vi "Disabled - Auton Script System (SubVI).vi"(8 "Alliance Color Input":string, 9 "Reload File Names":bool, 10 "Down File":bool, 11 "Up File":bool) -> (0 "error out":errorcluster, 1 "Files Reloaded":bool, 2 "Alliance Color":string, 3 "all rows":dbl[][](array[numeric]), 4 "File Name":string="_Do Nothing_.pi", 5 "File Names":string[](array[string]))   [LabVIEW 2020]
panel:
  in  "Computer Path":string="C:\\Users\\Pulsar\\Desktop\\FIRST 2012\\Autonomous\\1718 Read Auton Files\\"
  in  "Robot Path":string="/home/lvuser/Auton Scripts/"
  # "Select and Load Autonomous Mode"
  # "Controls"
  # "Indicators"
  # "Outputs"
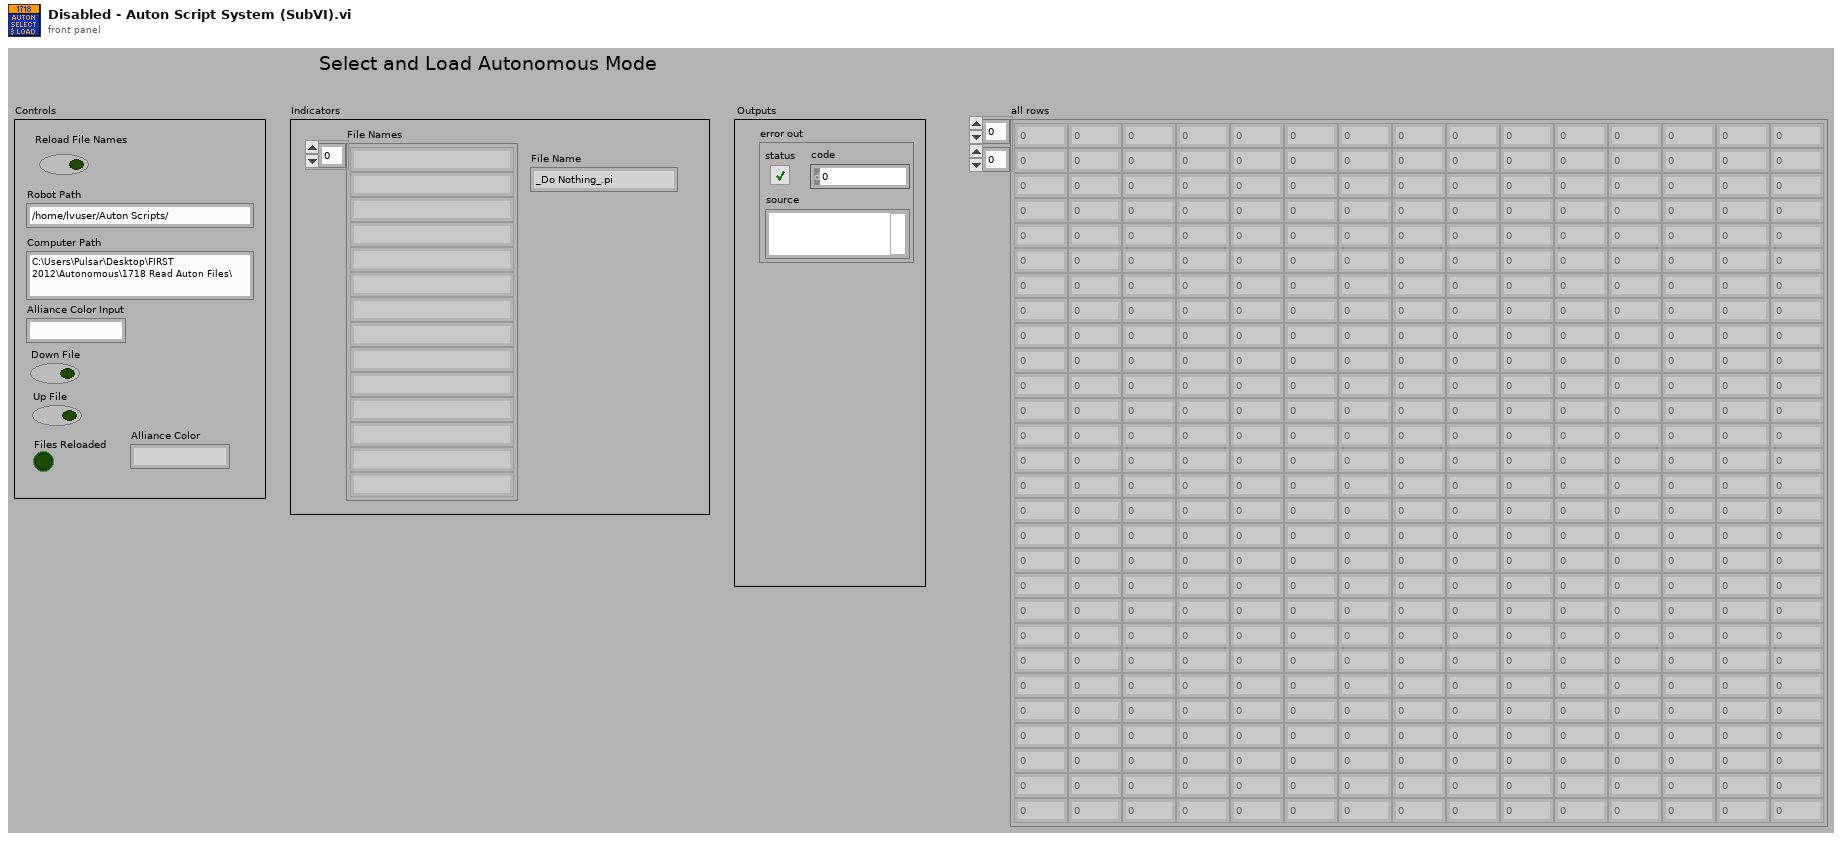
[diagram p1: front panel]
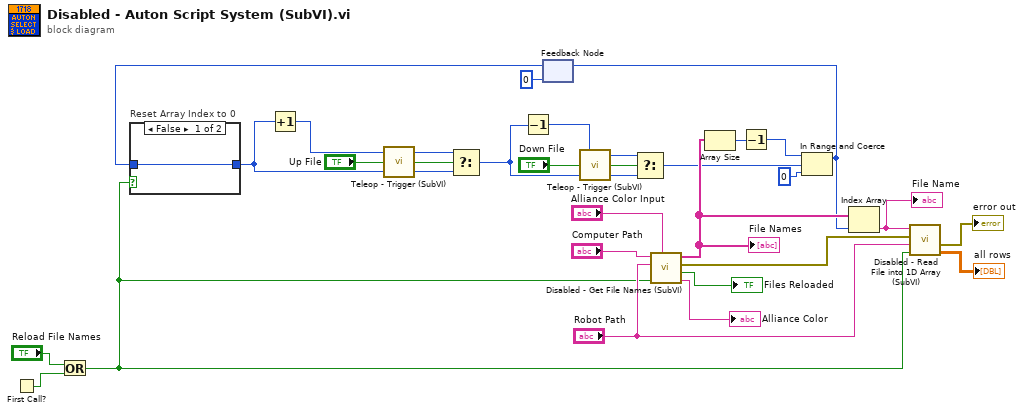
[diagram p0: block diagram]
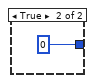
[diagram p2: hidden frame]
diagram:
  n1 = First Call?() -> (First Call?: T/F=w18:bool)
  n2 = Or(x="Reload File Names", y=w18) -> (x .or. y?=w16:bool)
  n3 = call "Teleop - Trigger (SubVI).vi"("Trigger"="Up File") -> ("Trigger Output"=w4:bool)
  n4 = feedback #1(0) -> (w11:i32)
  n5 = case "Reset Array Index to 0" shown="False" w16 {
    tunnel: [w29 0] -> w10
    tunnel: w11 -> [w29 _]
    frame False {
    }
    frame True {
    }
  }
  n6 = Increment(x=w10) -> (x+1=w14:i32)
  n7 = Select(t=w14, s=w4, f=w10) -> (s? t:f=w12:i32)
  n8 = Decrement(x=w12) -> (x-1=w13:i32)
  n9 = call "Teleop - Trigger (SubVI).vi"("Trigger"="Down File") -> ("Trigger Output"=w2:bool)
  n10 = Select(t=w13, s=w2, f=w12) -> (s? t:f=w9:i32)
  n11 = call "Disabled - Get File Names (SubVI).vi"("Alliance Color Input"="Alliance Color Input", "Reload File Names"=w16, "Robot Path"="Robot Path", "Computer Path"="Computer Path") -> ("Alliance Color"=→"Alliance Color":string, "Files Reloaded"=→"Files Reloaded":bool, "error out"=w6:errorcluster, "File Name Array"=w25:string[])  [unwired: 1 in]
  "File Names" <- w25
  n12 = Array Size(array=w25) -> (size(s)=w26:i32)
  n13 = Decrement(x=w26) -> (x-1=w21:i32)
  n14 = In Range and Coerce(upper limit=w21, x=w9, lower limit=0) -> (coerced(x)=w20:i32)  [unwired: 1 out]
  n15 = feedback-in #1(w20) -> ()
  n16 = Index Array(array=w25, index=w20) -> (element=w23:string)
  "File Name" <- w23
  n17 = call "Disabled - Read File into 1D Array (SubVI).vi"("Reload"=w16, "Path"="Robot Path", "error in"=w6, "File Name"=w23) -> ("all rows"=→"all rows":dbl[][], "error out"=→"error out":errorcluster)  [unwired: 1 in, 1 out]
